vi "global.vi"() -> ()   [LabVIEW 2014]
panel:
  out "g1":dbl
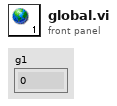
[diagram p1: front panel]
diagram:
